vi "Get Data from File.vi"(0 "VI Ref":refnum<vi>, 5 "Data Cluster In":T1={"Selected File"=path "", "Full Text File"=[], "Data Array"=[], "Times Array"=[], "Sensor Array"=[], "Subset Array"=[], "Smoothness Values"=[], "Sensor Select 1"=refnum, "Sensor Select 2"=refnum, "Sensor Select 3"=refnum, "Sensor Select 4"=refnum, "Start Times"=[], "End Times"=[], "Cursor List"=[{"Name"="Event Marker          ", "Color"=16777200, "Style"=0, "Point Style"=0, "Name Visible"=FALSE, "Allow Drag"=FALSE, "Cursor Mode"=0, "Plot"=0, "Index"=0, "Position"={"X"=4.0, "Y"=1.0}, "X Scale"=0, "Y Scale"=0, "Watch Plots"=[], "Watch All Plots"=FALSE, "Plot Area"=0, "Label Offset"={"X"=-50.0, "Y"=150.0}}, {"Name"="Upper Sensor", "Color"=13816500, "Style"=6, "Point Style"=0, "Name Visible"=FALSE, "Allow Drag"=FALSE, "Cursor Mode"=0, "Plot"=0, "Index"=0, "Position"={"X"=-1.0, "Y"=5.0}, "X Scale"=0, "Y Scale"=0, "Watch Plots"=[], "Watch All Plots"=FALSE, "Plot Area"=0, "Label Offset"={"X"=0.0, "Y"=0.0}}, {"Name"="Lower Sensor", "Color"=13816500, "Style"=6, "Point Style"=0, "Name Visible"=FALSE, "Allow Drag"=FALSE, "Cursor Mode"=0, "Plot"=0, "Index"=0, "Position"={"X"=-1.0, "Y"=30.0}, "X Scale"=0, "Y Scale"=0, "Watch Plots"=[], "Watch All Plots"=FALSE, "Plot Area"=0, "Label Offset"={"X"=0.0, "Y"=0.0}}], "Listbox 1"=refnum, "Listbox 2"=refnum, "Listbox 3"=refnum, "Listbox 4"=refnum, "Labels"=["Why", "is", "this", "still", "not", "built", "into", "Labview?", "This", "is", "shameful."], "Event Array"=[], "Event Names"=[], "Event Times"=[], "Save Plot Button"=refnum, "Sensor Plot Refs"=[], "Selected Event (Title)"="", "Upper Cursor"=0.0, "Lower Cursor"=0.0, "Z Max"=0.0, "Z Min"=0.0}, 11 "error in (no error)":errorcluster) -> (3 "Has Annotations?":bool, 4 "File Name":string, 6 "Data Cluster Out":T1={"Selected File"=path "", "Full Text File"=[], "Data Array"=[], "Times Array"=[], "Sensor Array"=[], "Subset Array"=[], "Smoothness Values"=[], "Sensor Select 1"=refnum, "Sensor Select 2"=refnum, "Sensor Select 3"=refnum, "Sensor Select 4"=refnum, "Start Times"=[], "End Times"=[], "Cursor List"=[{"Name"="Event Marker          ", "Color"=16777200, "Style"=0, "Point Style"=0, "Name Visible"=FALSE, "Allow Drag"=FALSE, "Cursor Mode"=0, "Plot"=0, "Index"=0, "Position"={"X"=4.0, "Y"=1.0}, "X Scale"=0, "Y Scale"=0, "Watch Plots"=[], "Watch All Plots"=FALSE, "Plot Area"=0, "Label Offset"={"X"=-50.0, "Y"=150.0}}, {"Name"="Upper Sensor", "Color"=13816500, "Style"=6, "Point Style"=0, "Name Visible"=FALSE, "Allow Drag"=FALSE, "Cursor Mode"=0, "Plot"=0, "Index"=0, "Position"={"X"=-1.0, "Y"=5.0}, "X Scale"=0, "Y Scale"=0, "Watch Plots"=[], "Watch All Plots"=FALSE, "Plot Area"=0, "Label Offset"={"X"=0.0, "Y"=0.0}}, {"Name"="Lower Sensor", "Color"=13816500, "Style"=6, "Point Style"=0, "Name Visible"=FALSE, "Allow Drag"=FALSE, "Cursor Mode"=0, "Plot"=0, "Index"=0, "Position"={"X"=-1.0, "Y"=30.0}, "X Scale"=0, "Y Scale"=0, "Watch Plots"=[], "Watch All Plots"=FALSE, "Plot Area"=0, "Label Offset"={"X"=0.0, "Y"=0.0}}], "Listbox 1"=refnum, "Listbox 2"=refnum, "Listbox 3"=refnum, "Listbox 4"=refnum, "Labels"=["Why", "is", "this", "still", "not", "built", "into", "Labview?", "This", "is", "shameful."], "Event Array"=[], "Event Names"=[], "Event Times"=[], "Save Plot Button"=refnum, "Sensor Plot Refs"=[], "Selected Event (Title)"="", "Upper Cursor"=0.0, "Lower Cursor"=0.0, "Z Max"=0.0, "Z Min"=0.0}, 8 "Subject Group":string, 10 "Subject Number":string, 14 "Has Annotations":string, 15 "error out":errorcluster)   [LabVIEW 2020]
uses:
  Controls/DataCluster.ctl
  <vilib>/Utility/miscctls.llb/LVCursorListTypeDef.ctl
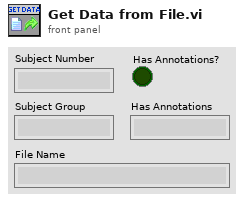
[diagram p1: front panel]
types:
  T1 = typedef "DataCluster.ctl" = cluster{"Selected File":path, "Full Text File":string[][], "Data Array":dbl[][], "Times Array":dbl[], "Sensor Array":dbl[], "Subset Array":dbl[][], "Smoothness Values":dbl[], "Sensor Select 1":refnum<vi>, "Sensor Select 2":refnum<vi>, "Sensor Select 3":refnum<vi>, "Sensor Select 4":refnum<vi>, "Start Times":dbl[], "End Times":dbl[], "Cursor List":T2, "Listbox 1":refnum<vi>, "Listbox 2":refnum<vi>, "Listbox 3":refnum<vi>, "Listbox 4":refnum<vi>, "Labels":string[], "Event Array":dbl[][], "Event Names":string[], "Event Times":dbl[], "Save Plot Button":refnum<vi>, "Sensor Plot Refs":refnum<vi>[], "Selected Event (Title)":string, "Upper Cursor":dbl, "Lower Cursor":dbl, "Z Max":dbl, "Z Min":dbl}
  T2 = typedef "LVCursorListTypeDef.ctl" = cluster{"Name":string, "Color":u32, "Style":u8, "Point Style":u8, "Name Visible":bool, "Allow Drag":bool, "Cursor Mode":u32, "Plot":i32, "Index":i32, "Position":cluster{"X":dbl, "Y":dbl}, "X Scale":u32, "Y Scale":u32, "Watch Plots":i32[], "Watch All Plots":bool, "Plot Area":i32, "Label Offset":cluster{"X":dbl, "Y":dbl}}[]
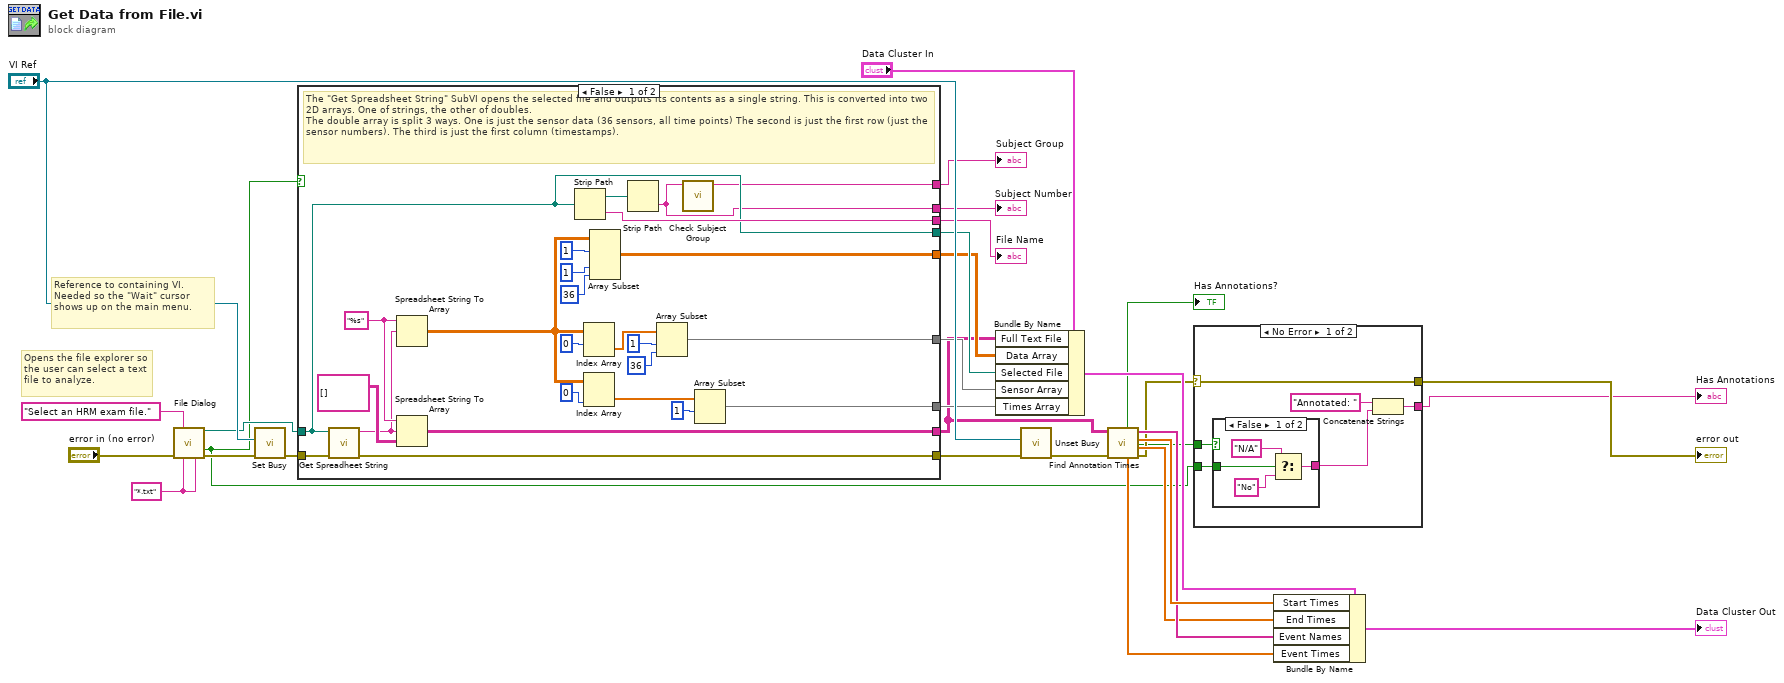
[diagram p0: block diagram]
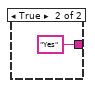
[diagram p2: hidden frame]
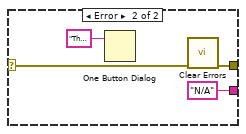
[diagram p3: hidden frame]
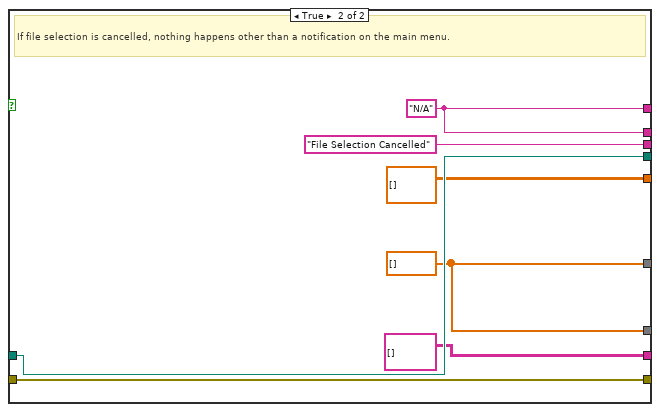
[diagram p4: hidden frame]
diagram:
  w9 = "*.txt" ("pattern label")
  # "Opens the file explorer so the user can select a text file to analyze."
  # "Reference to containing VI. Needed so the \"Wait\" cursor shows up on the main menu."
  n1 = call "File Dialog"("prompt"="Select an HRM exam file.", "error in"="error in (no error)", "pattern (all files)"=w9, "pattern label"=w9) -> ("selected path"=w21:path, "cancelled"=w2:bool, "error out"=w26:errorcluster)  [unwired: 8 in, 1 out]
  n2 = call <vilib>:"Set Busy.vi"("error in (no error)"=w26, "VI reference (current VI)"="VI Ref") -> ("error out"=w27:errorcluster)  [unwired: 8 in, 1 out]
  n3 = case shown="False" w2 {
    tunnel: w27 -> [w34 w61]
    tunnel: w21 -> [w35 w60]
    tunnel: [w50 dbl[][] []] -> w22
    tunnel: [w33 w61] -> w28
    tunnel: [w35 w60] -> w25
    tunnel: [w42 w59] -> w23
    tunnel: [w47 w59] -> w24
    tunnel: [w38 string[][] []] -> w14
    tunnel: [w37 "File Selection Cancelled"] -> w19
    tunnel: [w31 w55] -> w18
    tunnel: [w30 w55] -> w17
    frame False {
      w40 = "%s" ("format string")
      # "The \"Get Spreadsheet String\" SubVI opens the selected file and outputs its contents as a single string. This is converted into two 2D arrays. One of strings, the other of doubles. \nThe double array is split 3 ways. One is just the sensor data (36 sensors, all time points) The second is just the first row (just the sensor numbers). The third is just the first column (timestamps)."
      n4 = call "Get Spreadheet String.vi"("error in (no error)"=w34, "File Path"=w35) -> ("error out"=w33:errorcluster, "Spreadsheet String"=w32:string)  [unwired: 8 in]
      n5 = Spreadsheet String To Array(format string=w40, spreadsheet string=w32) -> (array=w41:dbl[][])  [unwired: 2 in]
      n6 = Spreadsheet String To Array(format string=w40, spreadsheet string=w32, array type (2D Dbl)=string[][] []) -> (array=w38:string[][])  [unwired: 1 in]
      n7 = Strip Path(path=w35) -> (stripped path=w36:path, name=w37:string)
      n8 = Index Array(array=w41, index (row)=0) -> (element=w48:dbl[])  [unwired: 1 in]
      n9 = Index Array(array=w41, index (col)=0 ("disabled index (col)")) -> (element=w43:dbl[])  [unwired: 1 in]
      n10 = Array Subset(array=w41, index (row)=1 ("index"), index (col)=1 ("index"), length (col)=36 ("length")) -> (w50:dbl[][])  [unwired: 1 in]
      n11 = Strip Path(path=w36) -> (name=w31:string)  [unwired: 1 out]
      n12 = Array Subset(array=w48, index=1, length=36) -> (w47:dbl[])
      n13 = call "Check Subject Group.vi"("Subject Number"=w31) -> ("Group"=w30:string)  [unwired: 10 in]
      n14 = Array Subset(array=w43, index=1) -> (w42:dbl[])  [unwired: 1 in]
    }
    frame True {
      w55 = "N/A" ("name")
      w59 = dbl[] []
      # "If file selection is cancelled, nothing happens other than a notification on the main menu."
    }
  }
  "File Name" <- w19
  "Subject Number" <- w18
  "Subject Group" <- w17
  n15 = Bundle By Name(cluster="Data Cluster In", "Full Text File"=w14, "Data Array"=w22, "Selected File"=w25, "Sensor Array"=w24, "Times Array"=w23) -> (w13:T1)
  n16 = call <vilib>:"Unset Busy.vi"("error in (no error)"=w28, "VI reference (current VI)"="VI Ref") -> ("error out"=w6:errorcluster)  [unwired: 9 in]
  n17 = call "Find Annotation Times.vi"("error in"=w6, "Full Text String Array"=w14) -> ("error out"=w5:errorcluster, "End Times"=w12:dbl[], "Start Times"=w16:dbl[], "Event Names"=w15:string[], "Event Times"=w7:dbl[], "Has Annotations?"=w3:bool)  [unwired: 4 in]
  "Has Annotations?" <- w3
  n18 = case shown="No Error" w5 {
    selector: w5 -> [w67 w75]
    tunnel: [w67 w74] -> w4
    tunnel: w3 -> [w64 _]
    tunnel: w2 -> [w63 _]
    tunnel: [w62 "N/A"] -> w1
    frame No Error {
      n19 = case shown="False" w64 {
        tunnel: [w70 "Yes"] -> w66
        tunnel: w63 -> [w71 _]
        frame False {
          n20 = Select(t="N/A" ("f"), s=w71, f="No") -> (s? t:f=w70:string)
        }
        frame True {
        }
      }
      n21 = Concatenate Strings("Annotated: " ("string"), w66) -> (w62:string)
    }
    frame Error {
      n22 = One Button Dialog(message="That was not an exam file.") -> ()  [unwired: 1 in, 1 out]
      n23 = call <vilib>:"Clear Errors.vi"("error in (no error)"=w75) -> ("error out"=w74:errorcluster)  [unwired: 5 in, 1 out]
    }
  }
  "error out" <- w4
  "Has Annotations" <- w1
  n24 = Bundle By Name(cluster=w13, "Start Times"=w16, "End Times"=w12, "Event Names"=w15, "Event Times"=w7) -> (→"Data Cluster Out":T1)
